vi "Get Port Id by handle.vi"(9 "port handle":u32, 10 "board handle":u32, 11 "hw_data in":T1) -> (0 "portId":u32, 1 "boardId":u32, 2 "key not found?":bool, 3 "hw_data out":T1)   [LabVIEW 2020, in "AIM664LV.lvlib"]
uses:
  AIM664LV.lvlib
  _controls/hwEntry_data.ctl
  _controls/hwEntryBoardHandleMap.ctl
  _controls/hwEntryBoardResource.ctl
  _controls/hwEntryPortResource.ctl
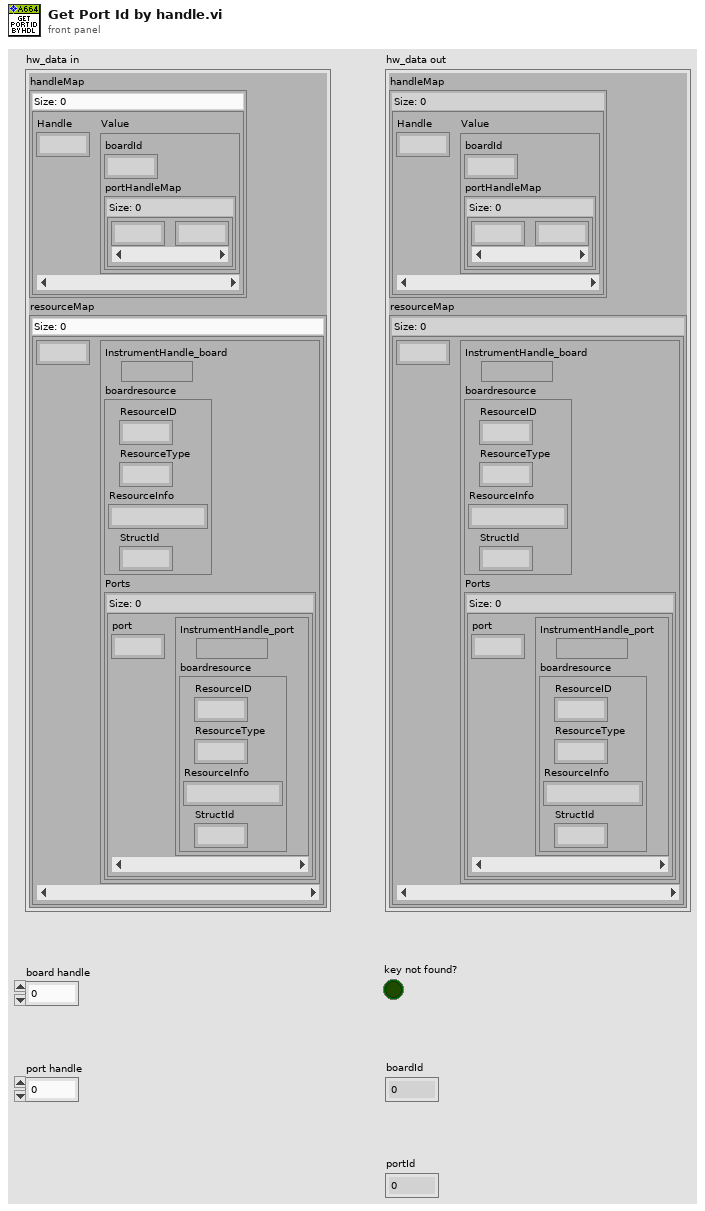
[diagram p1: front panel]
types:
  T1 = typedef "AIM664LV.lvlib/hwEntry_data.ctl" = cluster{"handleMap":map{u32, T2}, "resourceMap":map{u32, T3}}
  T2 = typedef "AIM664LV.lvlib/hwEntryBoardHandleMap.ctl" = cluster{"boardId":u32, "portHandleMap":map{u32, u32}}
  T3 = typedef "AIM664LV.lvlib/hwEntryBoardResource.ctl" = cluster{"InstrumentHandle_board":u32, "boardresource":cluster{"ResourceID":u32, "ResourceType":u32, "ResourceInfo":string, "StructId":u32}, "Ports":map{u32, T4}}
  T4 = typedef "AIM664LV.lvlib/hwEntryPortResource.ctl" = cluster{"InstrumentHandle_port":u32, "boardresource":cluster{"ResourceID":u32, "ResourceType":u32, "ResourceInfo":string, "StructId":u32}}
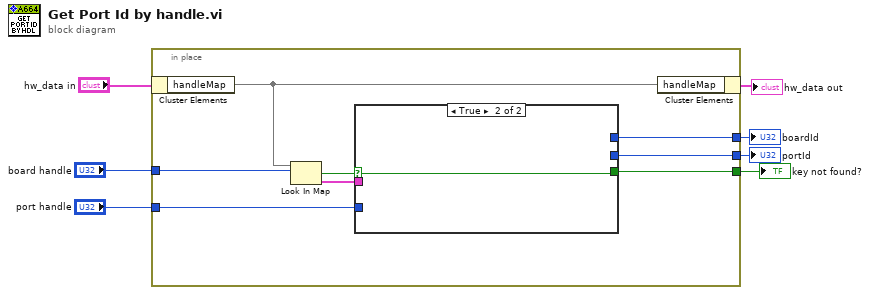
[diagram p0: block diagram]
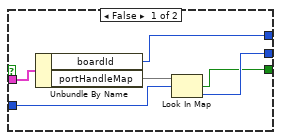
[diagram p2: hidden frame]
diagram:
  n1 = in-place {
    in-place-border: "board handle" -> [w15]
    in-place-border: [w11] -> w4
    in-place-border: "port handle" -> [w13]
    in-place-border: [w9] -> w2
    in-place-border: [w8] -> w1
    n2 = in-place-cluster #1("hw_data in") -> ("handleMap"=w10:map{u32, T2})
    n3 = Look In Map(map=w10, key=w15) -> (key not found?=w12:bool, value=w14:T2)  [unwired: 1 in]
    n4 = case shown="True" w12 {
      selector: w12 -> [_ w22]
      tunnel: w14 -> [w21 _]
      tunnel: w13 -> [w19 _]
      tunnel: [w17 w22] -> w11
      tunnel: [w18 _] -> w8
      tunnel: [w16 _] -> w9
      frame False {
        n5 = Unbundle By Name(w21) -> ("boardId"=w16:u32, "portHandleMap"=w20:map{u32, u32})
        n6 = Look In Map(map=w20, key=w19) -> (key not found?=w17:bool, value=w18:u32)  [unwired: 1 in]
      }
      frame True {
      }
    }
    n7 = in-place-cluster #1("handleMap"=w10) -> (→"hw_data out":T1)
  }
  "key not found?" <- w4
  "boardId" <- w2
  "portId" <- w1
